vi "AVS46.vi"(2 "Point #":i32, 3 "Instrument Address":refnum<visa-resource-name>) -> (0 "Stop":bool, 1 "Measurement":dbl[](array[numeric]) format="%.2f")   [LabVIEW 2019]
doc: "This VI reads the AVS resistance bridge.\nScott Hannahs, NHMFL-FSU, Nov 1993"
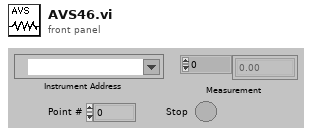
[diagram p1: front panel]
types:
  T1 = cluster{"Instrument":string, "ID Test String":string, "Terminator Character":string, u32, bool}
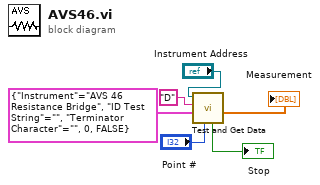
[diagram p0: block diagram]
diagram:
  n1 = call "Test and Get Data.vi"("Point #"="Point #", "Instrument Info"=T1 {"Instrument"="AVS 46 Resistance Bridge", "ID Test String"="", "Terminator Character"="", 0, FALSE}, "Command String"="D", "VISA Sesson"="Instrument Address") -> ("Measurement"=→"Measurement":dbl[], "Stop"=→"Stop":bool)  [unwired: 2 in, 3 out]
